vi "Read Numeric Text Props.vi"(8 "error in":errorcluster, 11 "Control in":refnum<vi>) -> (0 "error out":errorcluster, 2 "Numeric Text Props":T1, 3 "Control":refnum<vi>)   [LabVIEW 2020, in "VolatusGUIEditorCore.lvlib"]
uses:
  VolatusGUIEditorCore.lvlib
  Numeric Text Props.ctl
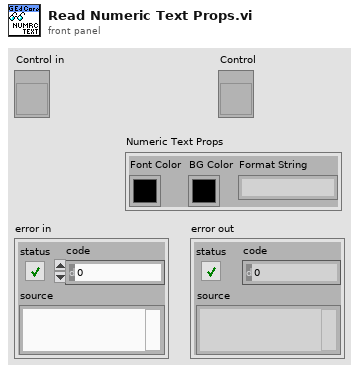
[diagram p1: front panel]
types:
  T1 = typedef "VolatusGUIEditorCore.lvlib/Numeric Text Props.ctl" = cluster{"Font Color":u32, "BG Color":u32, "Format String":string}
  T2 = cluster{"NumText.TextColor":u32, "NumText.BG Color":u32, "FormatString":string}
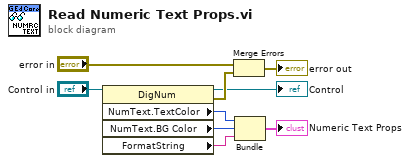
[diagram p0: block diagram]
diagram:
  n1 = property class="DigNum"(reference="Control in") -> (reference out=→"Control":refnum<vi>, error out=w9:errorcluster, "NumText.TextColor"=w4:u32, "NumText.BG Color"=w3:u32, "FormatString"=w2:string)  [unwired: 1 in]
  n2 = Merge Errors("error in", w9) -> (→"error out":errorcluster)
  n3 = Bundle("NumText.TextColor"=w4, "NumText.BG Color"=w3, "FormatString"=w2) -> (→"Numeric Text Props":T2)  [unwired: 1 in]
